vi "Go to Idle.vi"(8 "error in (no error)":errorcluster, 11 "Idle in":refnum<class "Idle.lvclass">) -> (0 "error out":errorcluster, 3 "Process State out":refnum<class "State Actor.lvclass">)   [LabVIEW 2025, in "Process States.lvlib" / "Idle.lvclass"]
doc: "This override disables entry behavior when entering the Idle state."
uses:
  Idle.lvclass
  <vilib>/ni/Actors/State Actor/State Actor/State Actor.lvclass
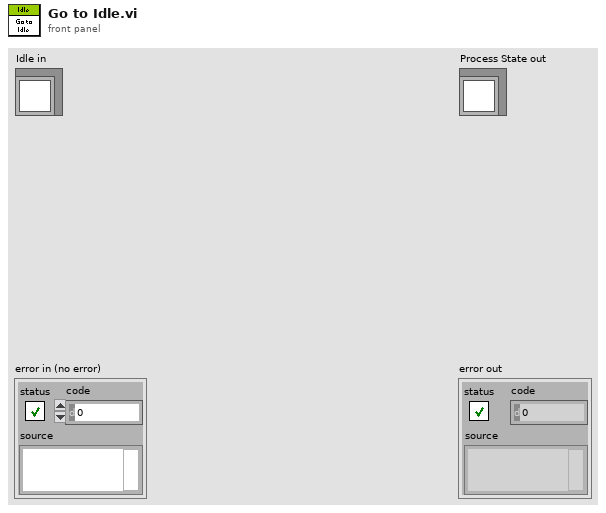
[diagram p1: front panel]
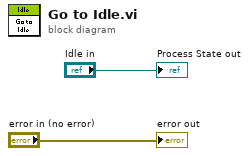
[diagram p0: block diagram]
diagram:
  "error out" <- "error in (no error)"
  "Process State out" <- "Idle in"
